vi "Wind Check.vi"(8 "error in (no error)":errorcluster, 10 "High Wind Speed":dbl, 11 "Current Wind Speed":dbl) -> (0 "error out":errorcluster, 1 "Wind Warning?":bool, 2 "Wind Warning Msg":string)   [LabVIEW 2010]
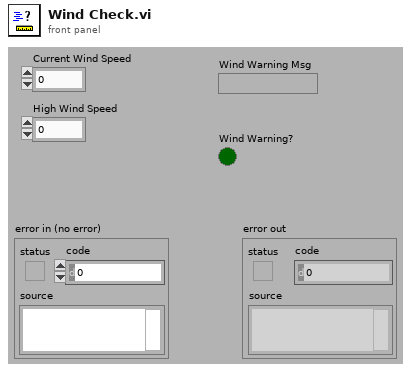
[diagram p1: front panel]
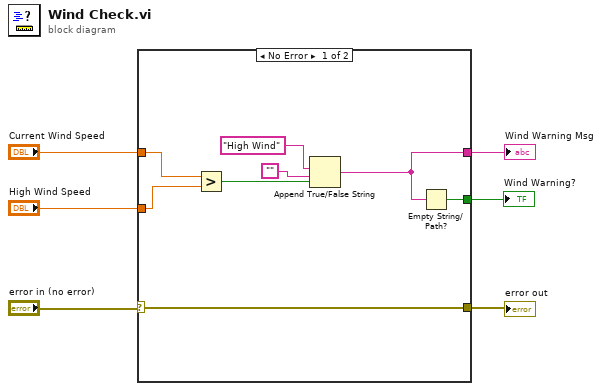
[diagram p0: block diagram]
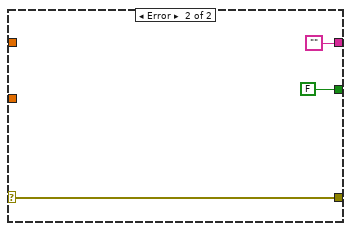
[diagram p2: hidden frame]
diagram:
  n1 = case shown="No Error" "error in (no error)" {
    selector: "error in (no error)" -> [w13 w17]
    tunnel: "Current Wind Speed" -> [w8 _]
    tunnel: "High Wind Speed" -> [w9 _]
    tunnel: [w7 ""] -> w4
    tunnel: [w14 FALSE] -> w3
    tunnel: [w13 w17] -> w1
    frame No Error {
      n2 = Greater?(x=w8, y=w9) -> (0:w10:bool)
      n3 = Append True/False String(1:w10, 2:"", 3:"High Wind") -> (0:w7:string)  [unwired: 1 out]
      n4 = Empty String/Path?(string/path=w7) -> (empty?=w14:bool)
    }
    frame Error {
    }
  }
  "Wind Warning Msg" <- w4
  "Wind Warning?" <- w3
  "error out" <- w1
